vi "driveEncoderConverter.vi"(7 "Conversion Direction":T2(ring), 10 "Gear Setting":T1, 11 "Input":dbl) -> (3 "Output":dbl format="%#_6f")   [LabVIEW 2018]
uses:
  driveShifterEnum.ctl
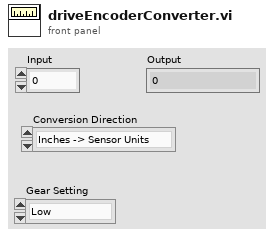
[diagram p1: front panel]
types:
  T1 = typedef "driveShifterEnum.ctl" = enum16{"Low", "High"}
  T2 = enum16{"Inches -> Sensor Units", "Sensor Units -> Inches"}
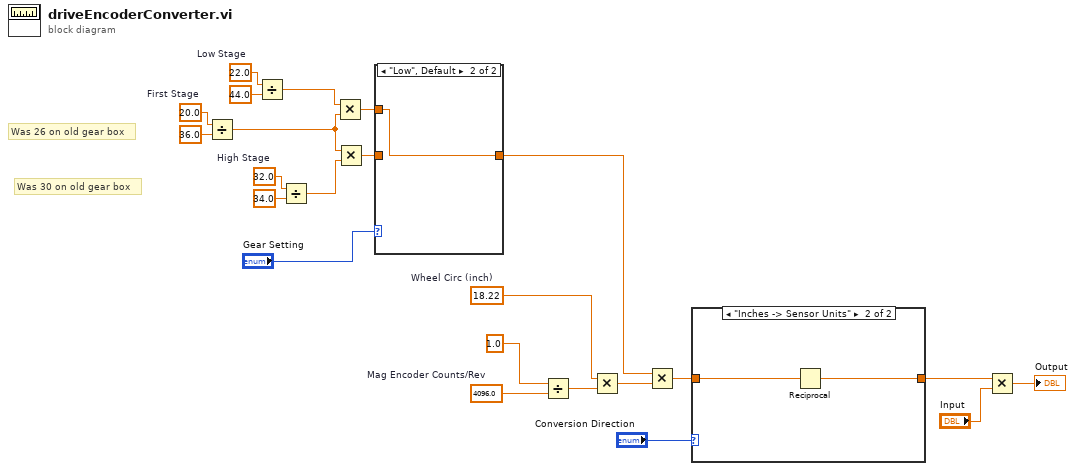
[diagram p0: block diagram]
diagram:
  w10 = 18.22  # Wheel Circ (inch)
  w6 = 4096.0  # Mag Encoder Counts/Rev
  w17 = 32.0  # High Stage
  w20 = 22.0  # Low Stage
  w23 = 20.0  # First Stage
  # "Was 30 on old gear box"
  # "Was 26 on old gear box"
  n1 = Divide(x=w23, y=36.0) -> (x/y=w18:dbl)
  n2 = Divide(x=w20, y=44.0) -> (x/y=w19:dbl)
  n3 = Divide(x=w17, y=34.0) -> (x/y=w15:dbl)
  n4 = Multiply(x=w19, y=w18) -> (x*y=w12:dbl)
  n5 = Multiply(x=w18, y=w15) -> (x*y=w13:dbl)
  n6 = case shown="\"Low\", Default" "Gear Setting" {
    tunnel: w13 -> [w24 _]
    tunnel: w12 -> [_ w25]
    tunnel: [w24 w25] -> w11
    frame "High" {
    }
    frame "Low", Default {
    }
  }
  n7 = Divide(x=1.0, y=w6) -> (x/y=w7:dbl)
  n8 = Multiply(x=w10, y=w7) -> (x*y=w14:dbl)
  n9 = Multiply(x=w11, y=w14) -> (x*y=w9:dbl)
  n10 = case shown="\"Inches -> Sensor Units\"" "Conversion Direction" {
    tunnel: w9 -> [w26 w28]
    tunnel: [w26 w27] -> w8
    frame "Sensor Units -> Inches" {
    }
    frame "Inches -> Sensor Units" {
      n11 = Reciprocal(x=w28) -> (1/x=w27:dbl)
    }
  }
  n12 = Multiply(x=w8, y="Input") -> (x*y=→"Output":dbl)
